vi "PB_Cburn_Stability.vi"(0 "Spectrum Parameters":T1={"Window 1 time (s)"=2e-05, "Window 2 time (s)"=1e-06, "Window 3 time (s) "=5e-08, "Window 4 time (s)"=2e-06, "Window 5 time (s)"=1e-07, "Window 6 time (s)"=5e-08, "Path to StabilityBurn"=path "C:/Users/Loncar/Desktop/ESR VIs - Srujan/Sam Kim/PB/StabilityBurn.exe", "Window 1 active channels"=[FALSE, TRUE], "Window 2 active channels"=[], "Window 3 active channels "=[FALSE, FALSE, TRUE], "Window 4 active channels"=[TRUE, FALSE, TRUE], "Window 5 active channels"=[FALSE, FALSE, TRUE], "Window 6 active channels"=[]}, 1 "# scans before track":i32=50, 2 "# steps":i32=50) -> (7 "String":string)   [LabVIEW 2012]
uses:
  Stability Window Parameters.ctl
panel:
  # "(outer loop)"
  # "(inner loop)"
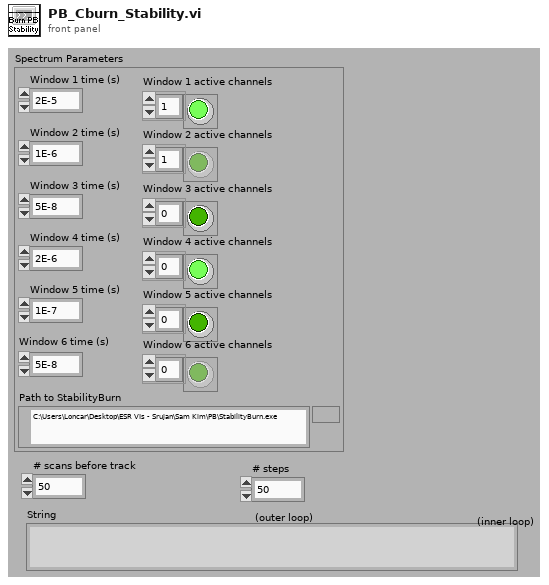
[diagram p1: front panel]
types:
  T1 = typedef "Stability Window Parameters.ctl" = cluster{"Window 1 time (s)":dbl, "Window 2 time (s)":dbl, "Window 3 time (s) ":dbl, "Window 4 time (s)":dbl, "Window 5 time (s)":dbl, "Window 6 time (s)":dbl, "Path to StabilityBurn":path, "Window 1 active channels":bool[], "Window 2 active channels":bool[], "Window 3 active channels ":bool[], "Window 4 active channels":bool[], "Window 5 active channels":bool[], "Window 6 active channels":bool[]}
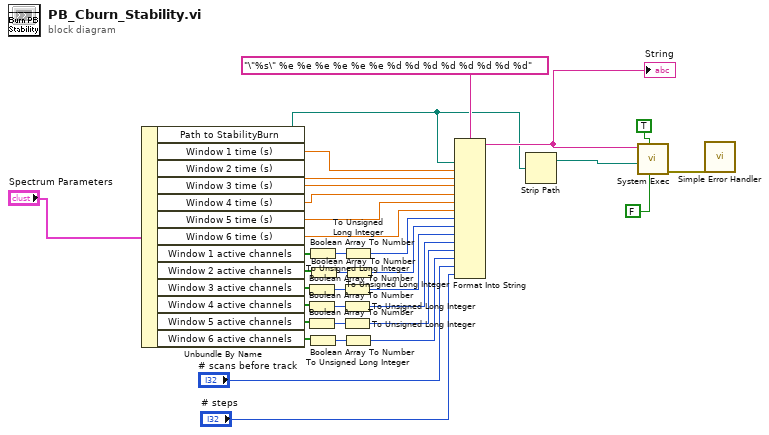
[diagram p0: block diagram]
diagram:
  n1 = Unbundle By Name("Spectrum Parameters") -> ("Path to StabilityBurn"=w22:path, "Window 1 time (s)"=w25:dbl, "Window 2 time (s)"=w24:dbl, "Window 3 time (s)"=w23:dbl, "Window 4 time (s)"=w20:dbl, "Window 5 time (s)"=w19:dbl, "Window 6 time (s)"=w18:dbl, "Window 1 active channels"=w16:bool[], "Window 2 active channels"=w14:bool[], "Window 3 active channels"=w13:bool[], "Window 4 active channels"=w11:bool[], "Window 5 active channels"=w8:bool[], "Window 6 active channels"=w4:bool[])
  n2 = Boolean Array To Number(Boolean array=w13) -> (number=w31:u32)
  n3 = Boolean Array To Number(Boolean array=w11) -> (number=w10:u32)
  n4 = Boolean Array To Number(Boolean array=w8) -> (number=w7:u32)
  n5 = Boolean Array To Number(Boolean array=w16) -> (number=w17:u32)
  n6 = Boolean Array To Number(Boolean array=w4) -> (number=w5:u32)
  n7 = Boolean Array To Number(Boolean array=w14) -> (number=w30:u32)
  n8 = To Unsigned Long Integer(number=w31) -> (unsigned 32bit integer=w12:u32)
  n9 = To Unsigned Long Integer(number=w10) -> (unsigned 32bit integer=w9:u32)
  n10 = To Unsigned Long Integer(number=w7) -> (unsigned 32bit integer=w6:u32)
  n11 = To Unsigned Long Integer(number=w17) -> (unsigned 32bit integer=w15:u32)
  n12 = To Unsigned Long Integer(number=w5) -> (unsigned 32bit integer=w3:u32)
  n13 = To Unsigned Long Integer(number=w30) -> (unsigned 32bit integer=w29:u32)
  n14 = Format Into String(format string="\"%s\" %e %e %e %e %e %e %d %d %d %d %d %d %d %d", w22, w25, w24, w23, w20, w19, w18, w15, w29, w12, w9, w6, w3, "# scans before track", "# steps") -> (resulting string=w27:string)  [unwired: 2 in, 1 out]
  "String" <- w27
  n15 = Strip Path(path=w22) -> (stripped path=w34:path)  [unwired: 1 out]
  n16 = call <vilib>:"System Exec.vi"("run minimized? (F)"=FALSE ("Wait until done"), "wait until completion? (T)"=TRUE ("Wait until done"), "working directory"=w34, "command line"=w27) -> ("error out"=w26:errorcluster)  [unwired: 4 in, 3 out]
  n17 = call <vilib>:"Simple Error Handler.vi"("error in (no error)"=w26) -> ()  [unwired: 4 in, 5 out]
